vi "lok_graf2.vi"() -> ()   [LabVIEW 2020]
uses:
  <vilib>/numeric/Random Number (Range) DBL.vi
panel:
  in  "stop":bool
  out "Waveform Chart":cluster{dbl, dbl}(graph)
  in  "Phase":dbl
  in  "Frekvence 2":dbl
  in  "Pocet vzorku":dbl
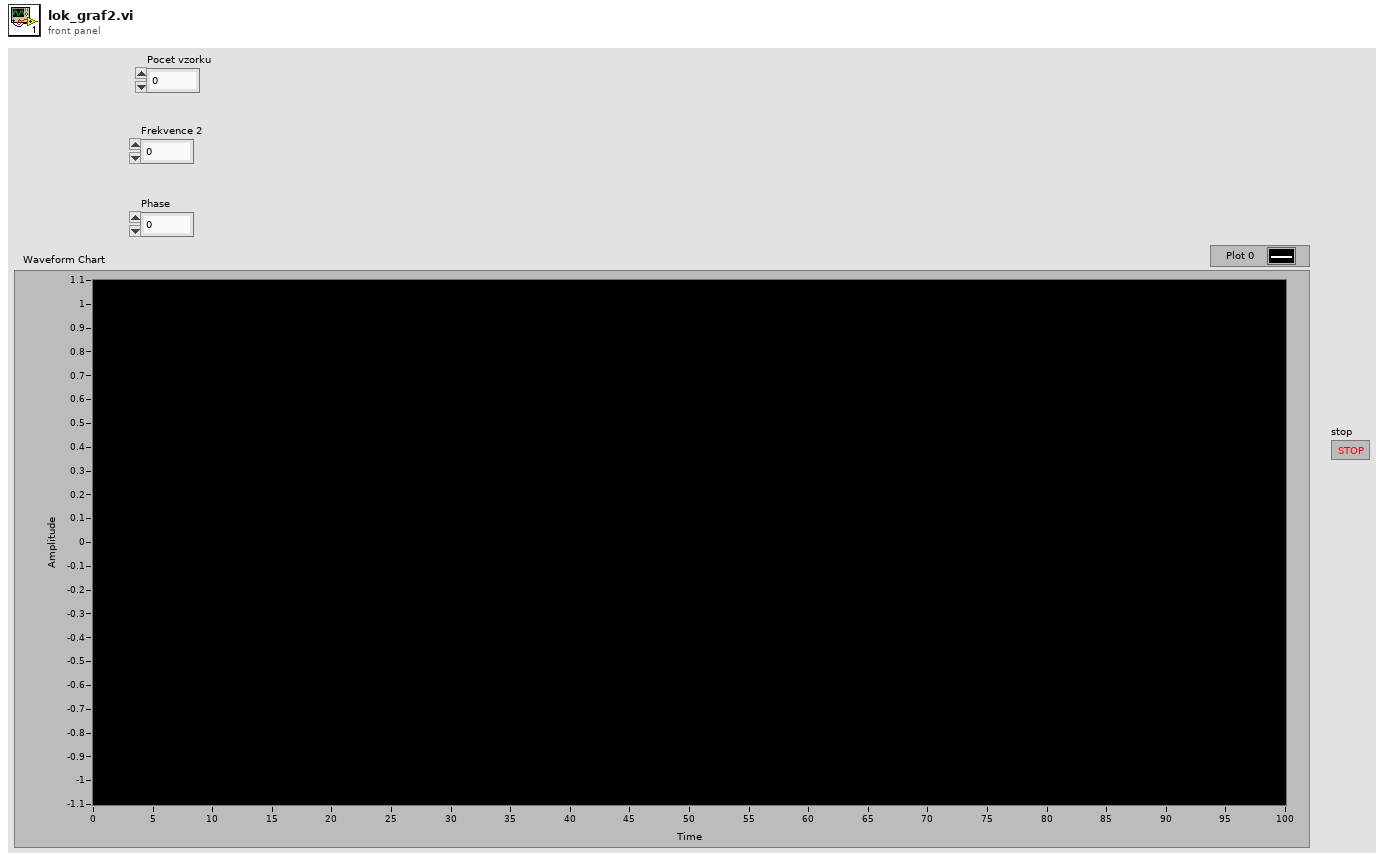
[diagram p1: front panel]
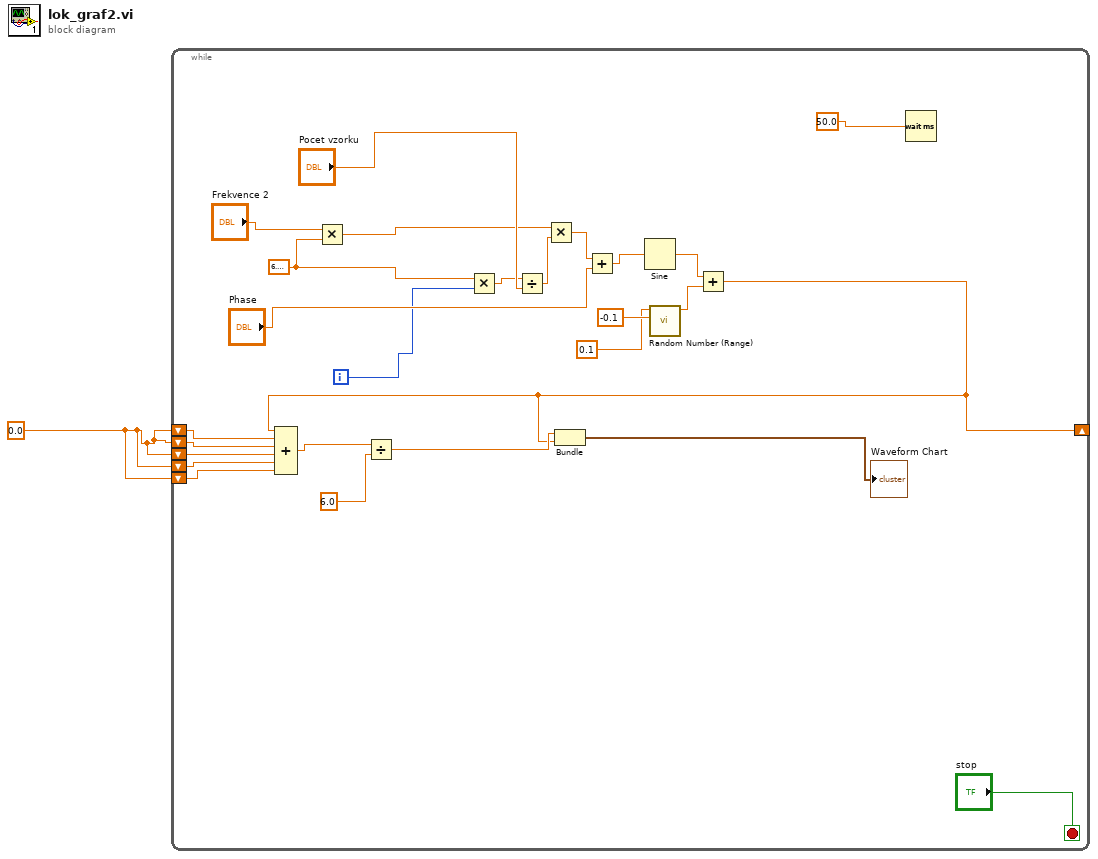
[diagram p0: block diagram]
diagram:
  w1 = 0.0
  n1 = while {
    shift-right: [w3] -> _
    shift-left: w1 -> [w11]
    shift-left: w1 -> [w10]
    shift-left: w1 -> [w9]
    shift-left: w1 -> [w8]
    shift-left: w1 -> [w7]
    i -> [w13]
    stop <- "stop" stop-if-true
    w23 = 6.283185307179586
    n2 = Multiply(x="Frekvence 2", y=w23) -> (x*y=w25:dbl)
    n3 = Multiply(x=w23, y=w13) -> (x*y=w20:dbl)
    n4 = Divide(x=w20, y="Pocet vzorku") -> (x/y=w19:dbl)
    n5 = Multiply(x=w25, y=w19) -> (x*y=w21:dbl)
    n6 = Add(x=w21, y="Phase") -> (x+y=w18:dbl)
    n7 = Sine(x=w18) -> (sin(x)=w17:dbl)
    n8 = call-poly <vilib>:"Random Number (Range).vi"("lower bound (0)"=-0.1, "upper bound (100)"=0.1) -> ("number"=w14:dbl)  [unwired: 9 in]
    n9 = Add(x=w17, y=w14) -> (x+y=w3:dbl)
    n10 = Compound Arithmetic op=ADD(w3, w11, w10, w9, w8, w7) -> (w6:dbl)
    n11 = Divide(x=w6, y=6.0) -> (x/y=w4:dbl)
    n12 = Bundle(w4, w3) -> (→"Waveform Chart":cluster{dbl, dbl})  [unwired: 1 in]
    n13 = Wait (ms)(milliseconds to wait=50.0) -> ()  [unwired: 1 out]
  }
